vi "Command Drop Tote.vi"(2 "Input Robot System Funtions":T1, 3 "Cmd Parameter 1":dbl, 4 "Cmd Parameter 2":dbl, 5 "Startup":bool) -> (0 "Output Robot System Functions":T1, 1 "Completed":bool)   [LabVIEW 2014]
uses:
  Subsystems VIs/Robot Commands.ctl
  Command Execution State.ctl
panel:
  # "Sample robot\ncontrol output.\nReplace with \nactual teleop \ncontrol signal \nstructure."
  # "Field Centric"
  # "Field Centric"
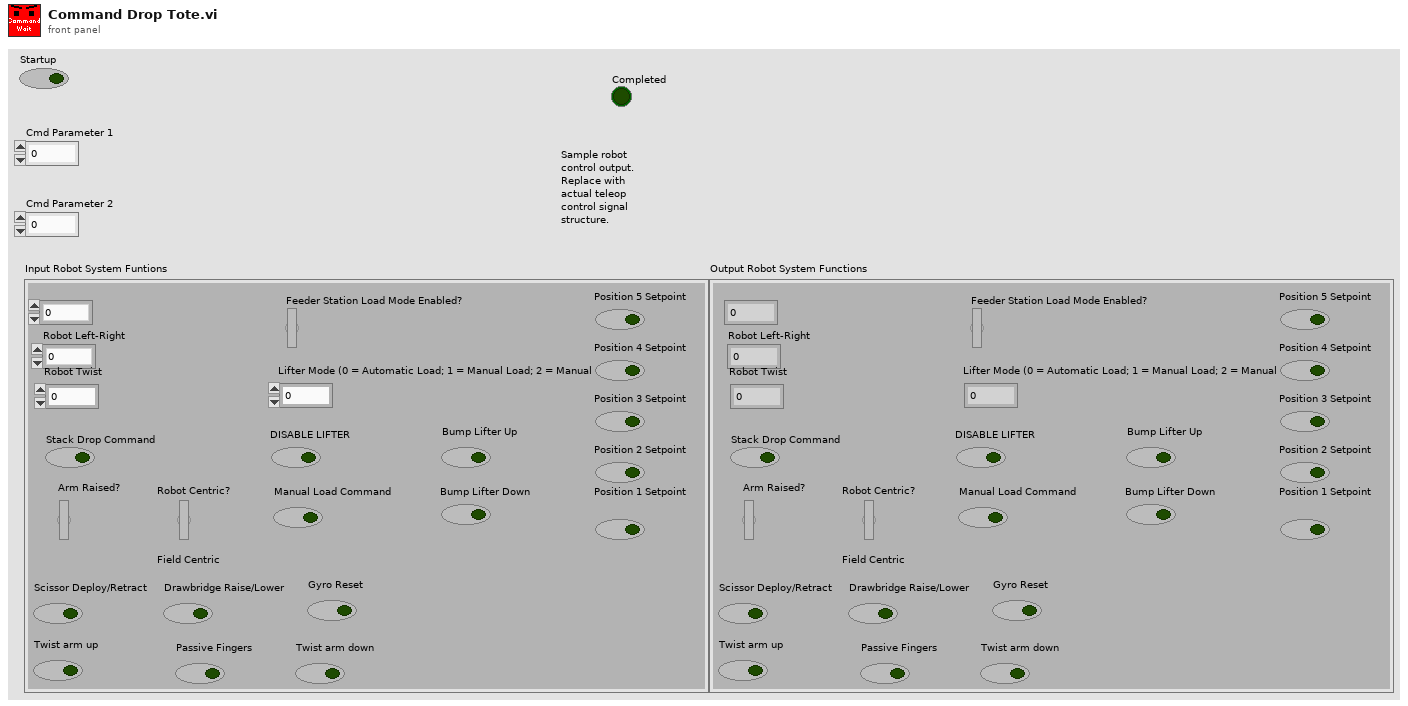
[diagram p1: front panel]
types:
  T1 = typedef "Robot Commands.ctl" = cluster{"Robot Forward-Reverse":dbl, "Robot Left-Right":dbl, "Robot Twist":dbl, "Feeder Station Load Mode Enabled?":bool, "Lifter Mode (0 = Automatic Load; 1 = Manual Load; 2 = Manual Override)":dbl, "Stack Drop Command":bool, "Arm Raised?":bool, "DISABLE LIFTER":bool, "Position 1 Setpoint":bool, "Position 2 Setpoint":bool, "Position 3 Setpoint":bool, "Position 4 Setpoint":bool, "Position 5 Setpoint":bool, "Bump Lifter Down":bool, "Bump Lifter Up":bool, "Manual Load Command":bool, "Robot Centric?":bool, "Scissor Deploy/Retract":bool, "Passive Fingers":bool, "Drawbridge Raise/Lower":bool, "Twist arm up":bool, "Gyro Reset":bool, "Twist arm down":bool}
  T2 = typedef "Command Execution State.ctl" = enum16{"Initialize", "Execute", "Finish"}
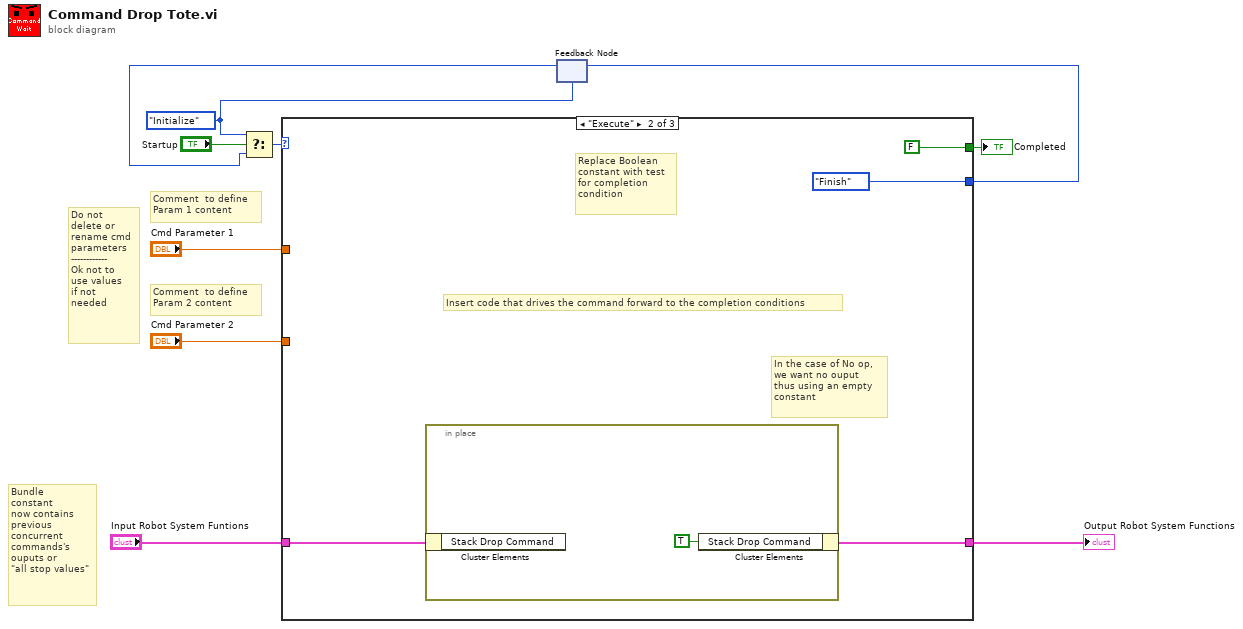
[diagram p0: block diagram]
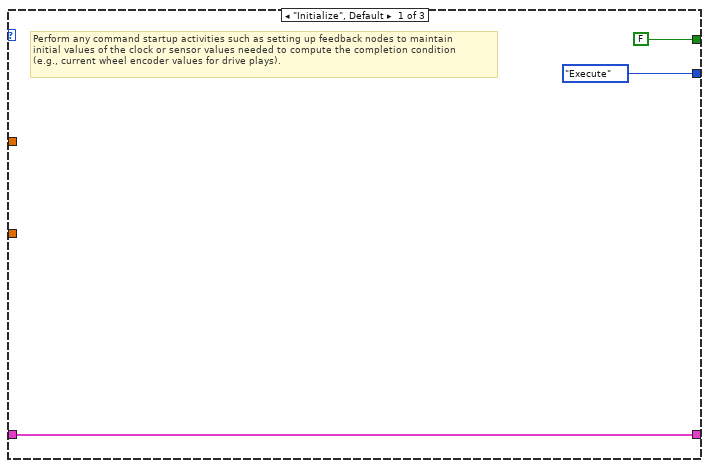
[diagram p2: hidden frame]
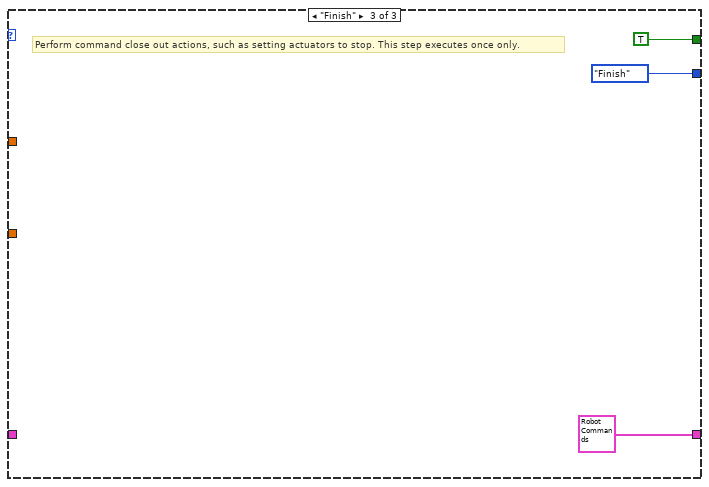
[diagram p3: hidden frame]
diagram:
  w5 = Command_Execution_State."Initialize" ("Play State")
  # "Bundle \nconstant\nnow contains\nprevious \nconcurrent\ncommands's\nouputs or\n\"all stop values\""
  # "Do not \ndelete or\nrename cmd\nparameters\n------------\nOk not to \nuse values\nif not \nneeded"
  # "Comment  to define\nParam 2 content"
  # "Comment  to define\nParam 1 content"
  n1 = feedback #1(w5) -> (w6:T2)
  n2 = Select(t=w5, s="Startup", f=w6) -> (s? t:f=w10:T2)
  n3 = case shown="\"Execute\"" w10 {
    tunnel: [FALSE FALSE TRUE] -> w8
    tunnel: [Command_Execution_State."Execute" ("Play State") Command_Execution_State."Finish" ("Play State") Command_Execution_State."Finish" ("f")] -> w7
    tunnel: "Cmd Parameter 1" -> [_ _ _]
    tunnel: "Cmd Parameter 2" -> [_ _ _]
    tunnel: [w11 w14 T1 {"Robot Forward-Reverse"=0.0, "Robot Left-Right"=0.0, "Robot Twist"=0.0, "Feeder Station Load Mode Enabled?"=FALSE, "Lifter Mode (0 = Automatic Load; 1 = Manual Load; 2 = Manual Override)"=0.0, "Stack Drop Command"=FALSE, "Arm Raised?"=FALSE, "DISABLE LIFTER"=FALSE, "Position 1 Setpoint"=FALSE, "Position 2 Setpoint"=FALSE, "Position 3 Setpoint"=FALSE, "Position 4 Setpoint"=FALSE, "Position 5 Setpoint"=FALSE, "Bump Lifter Down"=FALSE, "Bump Lifter Up"=FALSE, "Manual Load Command"=FALSE, "Robot Centric?"=FALSE, "Scissor Deploy/Retract"=FALSE, "Passive Fingers"=FALSE, "Drawbridge Raise/Lower"=FALSE, "Twist arm up"=FALSE, "Gyro Reset"=FALSE, "Twist arm down"=FALSE} ("Input Robot System Funtions")] -> w1
    tunnel: "Input Robot System Funtions" -> [w11 w15 _]
    frame "Initialize", Default {
      # "Perform any command startup activities such as setting up feedback nodes to maintain \ninitial values of the clock or sensor values needed to compute the completion condition\n(e.g., current wheel encoder values for drive plays)."
    }
    frame "Execute" {
      # "In the case of No op, \nwe want no ouput \nthus using an empty \nconstant"
      # "Replace Boolean\nconstant with test \nfor completion \ncondition"
      # "Insert code that drives the command forward to the completion conditions"
      n4 = in-place {
        n5 = in-place-cluster #2(w15) -> ()  [unwired: 1 out]
        n6 = in-place-cluster #2("Stack Drop Command"=TRUE) -> (w14:T1)
      }
    }
    frame "Finish" {
      # "Perform command close out actions, such as setting actuators to stop. This step executes once only."
    }
  }
  "Completed" <- w8
  "Output Robot System Functions" <- w1
  n7 = feedback-in #1(w7) -> ()
